vi "Slow Step.vi"(11 "time (ms)":u32) -> (3 "f":dbl)   [LabVIEW 2019, in "Instrument.Lockin.lvlib" / "Instrument.DAQ.lvclass"]
uses:
  Instrument.DAQ.lvclass
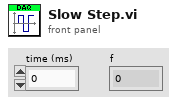
[diagram p1: front panel]
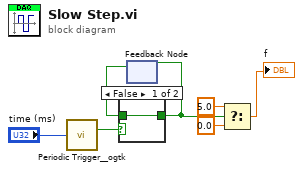
[diagram p0: block diagram]
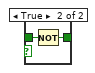
[diagram p2: hidden frame]
diagram:
  n1 = call <userlib>:"Periodic Trigger__ogtk.vi"("time (ms)"="time (ms)") -> ("Triggered"=w7:bool)  [unwired: 12 in, 2 out]
  n2 = feedback #1() -> (w5:bool)  [unwired: 1 in]
  n3 = case shown="False" w7 {
    tunnel: w5 -> [w8 w10]
    tunnel: [w8 w9] -> w6
    frame False {
    }
    frame True {
      n4 = Not(x=w10) -> (.not. x?=w9:bool)
    }
  }
  n5 = feedback-in #1(w6) -> ()
  n6 = Select(t=5.0, s=w6, f=0.0) -> (s? t:f=→"f":dbl)
